vi "UnitConversion.vi"(10 "Net Right Pulse":dbl, 11 "Net Left Pulse":dbl) -> (2 "X":dbl, 3 "Y":dbl)   [LabVIEW 2017]
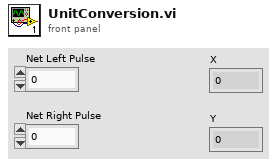
[diagram p1: front panel]
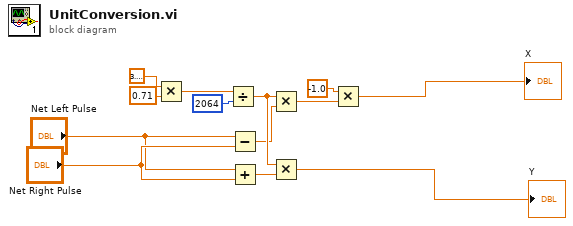
[diagram p0: block diagram]
diagram:
  n1 = Multiply(x=3.141592653589793, y=0.71) -> (x*y=w3:dbl)
  n2 = Divide(x=w3, y=2064) -> (x/y=w9:dbl)
  n3 = Subtract(x="Net Left Pulse", y="Net Right Pulse") -> (x-y=w8:dbl)
  n4 = Add(x="Net Left Pulse", y="Net Right Pulse") -> (x+y=w5:dbl)
  n5 = Multiply(x=w9, y=w8) -> (x*y=w11:dbl)
  n6 = Multiply(x=w9, y=w5) -> (x*y=→"Y":dbl)
  n7 = Multiply(x=-1.0, y=w11) -> (x*y=→"X":dbl)
